vi "Scan_Controller.vi"(4 "timeout (10msec)":u32=100, 5 "error in (no error)":errorcluster, 6 "Scan End":i32, 7 "Scan Start":i32, 8 "VISA resource name":refnum<visa-resource-name>) -> (0 "error out":errorcluster, 2 "Array":i32[](array[numeric]), 3 "VISA resource name out":refnum<visa-resource-name>)   [LabVIEW 2019, in "Faulhaber RS232.lvlib"]
uses:
  Faulhaber RS232.lvlib
  <vilib>/Instr/_visa.llb/VISA Configure Serial Port (Instr).vi
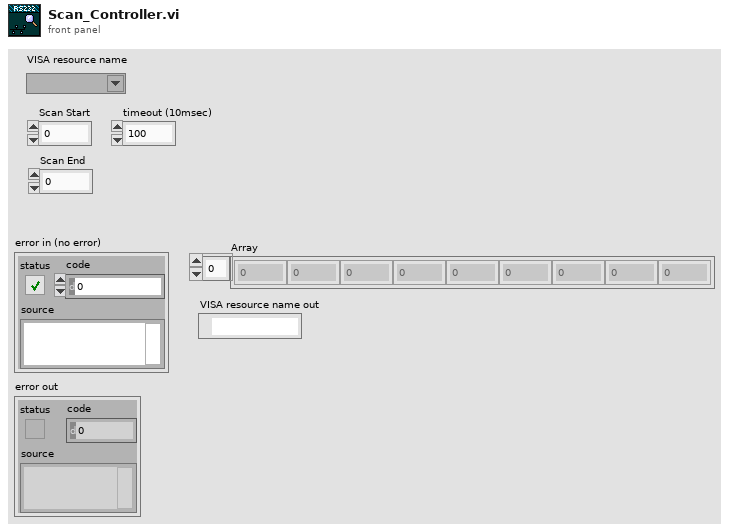
[diagram p1: front panel]
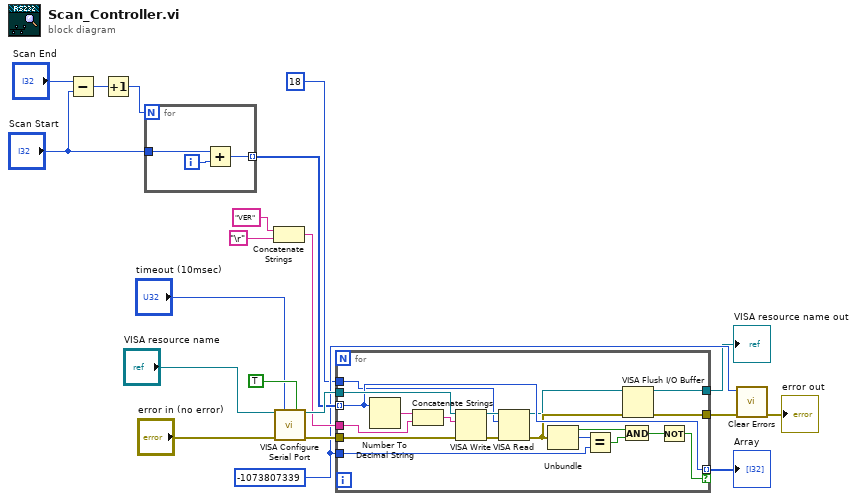
[diagram p0: block diagram]
diagram:
  w4 = -1073807339 ("y")
  n1 = Subtract(x="Scan End", y="Scan Start") -> (x-y=w19:i32)
  n2 = Increment(x=w19) -> (x+1=w18:i32)
  n3 = for {
    N: w18 -> [_]
    tunnel: "Scan Start" -> [w22]
    tunnel: [w21] -> w16 mode=indexing
    i -> [w23]
    n4 = Add(x=w22, y=w23) -> (x+y=w21:i32)
  }
  n5 = Concatenate Strings("VER", "\r") -> (w13:string)
  n6 = call-poly "VISA Configure Serial Port"("VISA resource name"="VISA resource name", "timeout (10sec)"="timeout (10msec)", "Enable Termination\nChar (T)"=TRUE ("Enable Termination\nChar (T)"), "error in (no error)"="error in (no error)") -> ("VISA resource name out"=w20:refnum<visa-resource-name>, "error out"=w10:errorcluster)  [unwired: 10 in]
  n7 = for {
    tunnel: w16 -> [w35] mode=indexing
    tunnel: w13 -> [w39]
    tunnel: [w35] -> w7 mode=indexing if=w25
    tunnel: w10 -> [w36]
    tunnel: [w27] -> w5
    tunnel: w4 -> [w26]
    tunnel: w20 -> [w42]
    tunnel: [w28] -> w2
    tunnel: u32 18 ("byte count") -> [w24]
    n8 = Number To Decimal String(number=w35) -> (decimal integer string=w40:string)  [unwired: 1 in]
    n9 = Concatenate Strings(w40, w39) -> (w38:string)
    n10 = VISA Write(VISA resource name=w42, write buffer=w38, error in (no error)=w36) -> (VISA resource name out=w41:refnum<visa-resource-name>, error out=w37:errorcluster)  [unwired: 1 out]
    n11 = VISA Read(VISA resource name=w41, byte count=w24, error in (no error)=w37) -> (VISA resource name out=w29:refnum<visa-resource-name>, error out=w30:errorcluster)  [unwired: 2 out]
    n12 = Unbundle(w30) -> ("status"=w31:bool, "code"=w34:i32)  [unwired: 1 out]
    n13 = Equal?(x=w34, y=w26) -> (x = y?=w33:bool)
    n14 = And(x=w31, y=w33) -> (x .and. y?=w32:bool)
    n15 = VISA Flush I/O Buffer(VISA resource name=w29, error in (no error)=w30) -> (VISA resource name out=w28:refnum<visa-resource-name>, error out=w27:errorcluster)  [unwired: 1 in]
    n16 = Not(x=w32) -> (.not. x?=w25:bool)
  }
  "Array" <- w7
  "VISA resource name out" <- w2
  n17 = call <vilib>:"Clear Errors.vi"("error in (no error)"=w5, "specific error code to clear (0: all)"=w4) -> ("error out"=→"error out":errorcluster)  [unwired: 4 in, 1 out]
